vi "InitBoard.vi"(9 "Board Color":u32(colorbox)=16728794, 10 "BoardSize":cluster{"X":i32, "Y":i32}) -> (0 "error out":errorcluster, 3 "SnakeGame out":refnum<class "Snake.lvclass">)   [LabVIEW 2021]
uses:
  Snake.lvclass
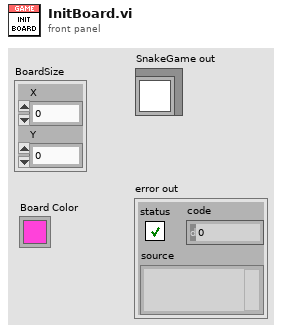
[diagram p1: front panel]
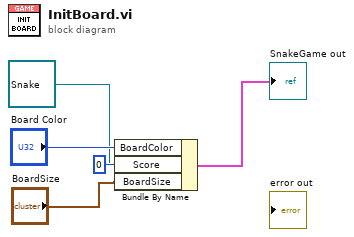
[diagram p0: block diagram]
diagram:
  n1 = Bundle By Name(cluster=refnum<class "Snake.lvclass"> refnum ("SnakeGame.lvclass"), "BoardColor"="Board Color", "Score"=u32 0, "BoardSize"="BoardSize") -> (→"SnakeGame out":cluster{})
